vi "Close.vi"(8 "error in (no error)":errorcluster, 11 "UndoObject in":refnum<class "UndoObject.lvclass">) -> (0 "error out":errorcluster)   [LabVIEW 2015, in "UndoLibrary.lvlib" / "UndoObject.lvclass"]
doc: "This VI destroys the references to store the values of the control."
uses:
  UndoObject.lvclass
  UndoObject.lvclass/UndoObject.ctl
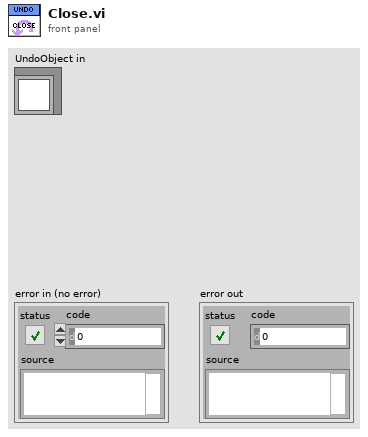
[diagram p1: front panel]
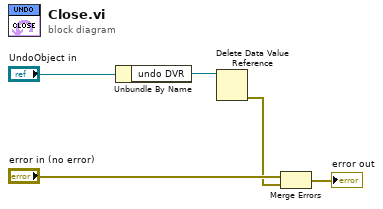
[diagram p0: block diagram]
diagram:
  n1 = Unbundle By Name("UndoObject in") -> ("undo DVR"=w2:refnum<data-value>)
  n2 = Delete Data Value Reference(data value reference=w2) -> (error out=w1:errorcluster)  [unwired: 1 in, 1 out]
  n3 = Merge Errors("error in (no error)", w1) -> (→"error out":errorcluster)
